vi "FlightRecorder.vi"   [LabVIEW 2014]
uses:
  <vilib>/Utility/file.llb/Write To Spreadsheet File (DBL).vi
  <vilib>/Utility/file.llb/Write To Spreadsheet File (string).vi
types:
  T1 = typedef "WPI_MotorControlDeviceRef.ctl" = cluster{"DeviceStatus":errorcluster, "Type":T2, "PWM":cluster{"Controller":T3, "PWM Channel":T4, "DeadBand":T5}, "CAN":cluster{"Device Number":u8, "Control Mode":T6, "Semaphore":T7, "Max Vout":dbl, "TalonSRX Control Mode":T8}, "Invert":bool, "TransformRef":T9, "InvTransformRef":T9}
  T2 = typedef "WPI_MotorControlType.ctl" = enum16{"PWM", "CAN", "CANTalonSRX"}
  T3 = typedef "FPGA_TypedefDigitalModule.ctl" = enum16{"Controller 1"}
  T4 = typedef "FPGA_DIOPWMChannel.ctl" = enum8{"PWM 0", "PWM 1", "PWM 2", "PWM 3", "PWM 4", "PWM 5", "PWM 6", "PWM 7", "PWM 8", "PWM 9", "PWM MXP 0", "PWM MXP 1", "PWM MXP 2", "PWM MXP 3", "PWM MXP 4", "PWM MXP 5", "PWM MXP 6", "PWM MXP 7", "PWM MXP 8", "PWM MXP 9", "Invalid"}
  T5 = typedef "WPI_PWMDeadband.ctl" = cluster{"Name":string, "maxPositivePwm":i32, "minPositivePwm":i32, "centerPwm":i32, "maxNegativePwm":i32, "minNegativePwm":i32, "angularRange":u16}
  T6 = typedef "WPI_CANJaguar_ControlMode.ctl" = enum8{"Percent VBus", "Current", "Speed", "Position", "Voltage"}
  T7 = typedef "Semaphore RefNum" = refnum<k1>
  T8 = typedef "WPI_CANTalonSRX_APIControlMode.ctl" = enum8{"Percent VBus", "Speed", "Position", "Slave", "Unchanged / Invalid"}
  T9 = typedef "WPI_PWMTransform_ConPane.ctl" = refnum<vi>
  T10 = typedef "WPI_CANTalonSRX_GlobalStatus.ctl" = cluster{"Applied Throttle":dbl, "Module Enabled":bool, "CAN Error":errorcluster, "Closed Loop Error":dbl, "Forward Limit Switch Closed":bool, "Reverse Limit Switch Closed":bool, "Sensor Position":dbl, "Sensor Velocity":dbl, "Current":dbl, "Sticky Fault - Over Temp":bool, "Sticky Fault - Under Voltage":bool, "Sticky Fault - Forward Limit":bool, "Sticky Fault - Reverse Limit":bool, "Sticky Fault - Forward Soft Limit":bool, "Sticky Fault - Reverse Soft Limit":bool, "Brake is Enabled":bool, "Encoder Position":dbl, "Encoder Velocity":dbl, "Encoder Index Count":dbl, "Encoder A Pin State":bool, "Encoder B Pin State":bool, "Encoder Index Pin State":bool, "Analog In":dbl, "Analog In Velocity":dbl, "Temperature (C)":dbl, "Battery Voltage":dbl}
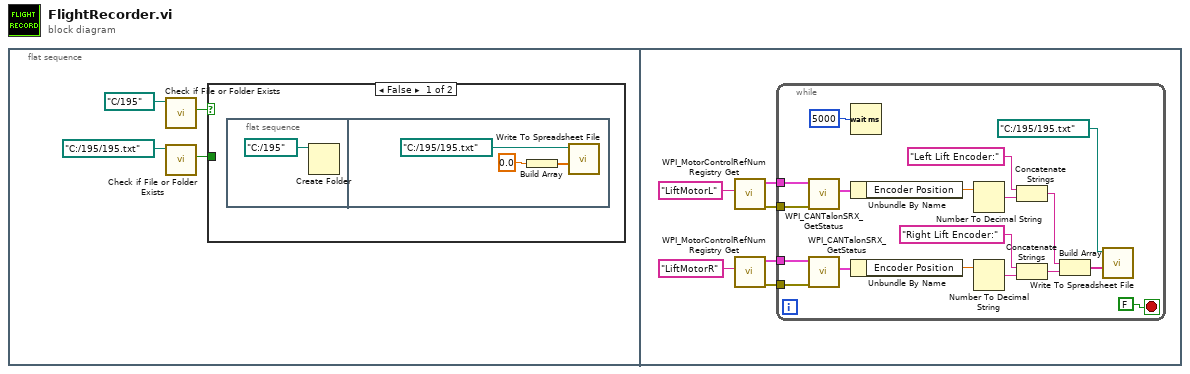
[diagram p0: block diagram]
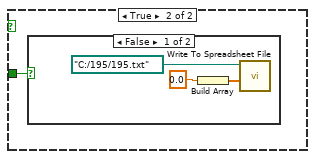
[diagram p2: hidden frame]
diagram:
  n1 = flat-sequence {
    frame #0 {
      n2 = call <vilib>:"Check if File or Folder Exists.vi"("path"=path "C:/195") -> ("file or folder exists?"=w3:bool)  [unwired: 8 in, 2 out]
      n3 = call <vilib>:"Check if File or Folder Exists.vi"("path"=path "/C:/195/195.txt") -> ("file or folder exists?"=w1:bool)  [unwired: 8 in, 2 out]
      n4 = case shown="False" w3 {
        tunnel: w1 -> [_ w9]
        frame False {
          n5 = flat-sequence {
            frame #0 {
              n6 = Create Folder(path (use dialog)=path "/C:/195") -> ()  [unwired: 2 in, 3 out]
            }
            frame #1 {
              n7 = Build Array(0.0 ("element")) -> (w7:dbl[])
              n8 = call-poly <vilib>:"Write To Spreadsheet File.vi"("1D data"=w7, "file path (dialog if empty)"=path "/C:/195/195.txt" ("file path (use dialog)")) -> ()  [unwired: 6 in, 1 out]
            }
          }
        }
        frame True {
          n9 = case shown="False" w9 {
            frame False {
              n10 = Build Array(0.0 ("element")) -> (w11:dbl[])
              n11 = call-poly <vilib>:"Write To Spreadsheet File.vi"("1D data"=w11, "file path (dialog if empty)"=path "/C:/195/195.txt" ("file path (use dialog)")) -> ()  [unwired: 6 in, 1 out]
            }
            frame True {
            }
          }
        }
      }
    }
    frame #1 {
      n12 = call <vilib>:"WPI_MotorControlRefNum Registry Get.vi"("refnum name"="LiftMotorL") -> ("error out"=w13:errorcluster, "MotorControlDevRef"=w14:T1)  [unwired: 9 in]
      n13 = call <vilib>:"WPI_MotorControlRefNum Registry Get.vi"("refnum name"="LiftMotorR") -> ("error out"=w16:errorcluster, "MotorControlDevRef"=w15:T1)  [unwired: 9 in]
      n14 = while {
        tunnel: w16 -> [w34]
        tunnel: w15 -> [w33]
        tunnel: w14 -> [w32]
        tunnel: w13 -> [w31]
        stop <- FALSE stop-if-true
        n15 = call <vilib>:"WPI_CANTalonSRX_GetStatus.vi"("error in (no error)"=w31, "CAN Talon SRX Ref"=w32) -> ("Talon SRX Status"=w30:T10)  [unwired: 7 in, 2 out]
        n16 = call <vilib>:"WPI_CANTalonSRX_GetStatus.vi"("error in (no error)"=w34, "CAN Talon SRX Ref"=w33) -> ("Talon SRX Status"=w29:T10)  [unwired: 7 in, 2 out]
        n17 = Wait (ms)(milliseconds to wait=u32 5000) -> ()  [unwired: 1 out]
        n18 = Unbundle By Name(w30) -> ("Encoder Position"=w27:dbl)
        n19 = Unbundle By Name(w29) -> ("Encoder Position"=w22:dbl)
        n20 = Number To Decimal String(number=w27) -> (decimal integer string=w26:string)  [unwired: 1 in]
        n21 = Number To Decimal String(number=w22) -> (decimal integer string=w24:string)  [unwired: 1 in]
        n22 = Concatenate Strings("Left Lift Encoder:" ("string"), w26) -> (w25:string)
        n23 = Concatenate Strings("Right Lift Encoder:" ("string"), w24) -> (w21:string)
        n24 = Build Array(w25, w21) -> (w20:string[])
        n25 = call-poly <vilib>:"Write To Spreadsheet File.vi"("1D data"=w20, "file path (dialog if empty)"=path "/C:/195/195.txt") -> ()  [unwired: 6 in, 1 out]
      }
    }
  }
